vi "MaskBoxToTipCoords.vi"(9 "manip 1 position":T1={"width x"=498.0, "height y"=180.0, "x offset"=32.0, "y offset"=116.0}, 11 "bounding rectangle":i32[](array[numeric])) -> (3 "user selected pipette tip (x,y)":i32[](array[numeric]))   [LabVIEW 2015]
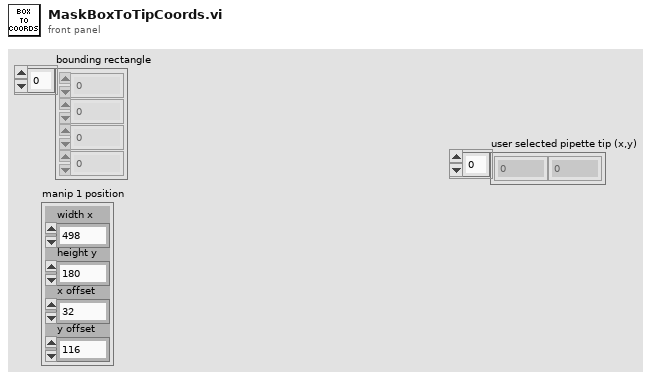
[diagram p1: front panel]
types:
  T1 = cluster{"width x":dbl, "height y":dbl, "x offset":dbl, "y offset":dbl}
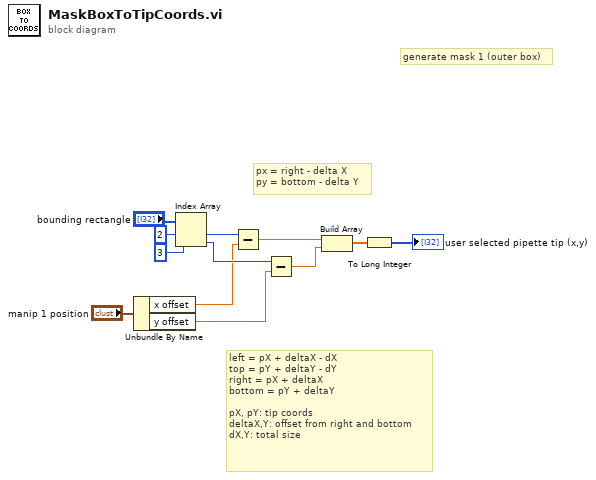
[diagram p0: block diagram]
diagram:
  # "px = right - delta X\npy = bottom - delta Y"
  # "left = pX + deltaX - dX\ntop = pY + deltaY - dY\nright = pX + deltaX\nbottom = pY + deltaY\n\npX, pY: tip coords\ndeltaX,Y: offset from right and bottom\ndX,Y: total size"
  # "generate mask 1 (outer box)"
  n1 = Unbundle By Name("manip 1 position") -> ("x offset"=w8:dbl, "y offset"=w7:dbl)
  n2 = Index Array(array="bounding rectangle", index #1=2 ("index"), index #2=3 ("index")) -> (element #1=w10:i32, element #2=w9:i32)
  n3 = Subtract(x=w10, y=w8) -> (x-y=w6:dbl)
  n4 = Subtract(x=w9, y=w7) -> (x-y=w5:dbl)
  n5 = Build Array(w6, w5) -> (w4:dbl[])
  n6 = To Long Integer(number=w4) -> (32bit integer=→"user selected pipette tip (x,y)":i32[])
